vi "output check.vi"() -> ()   [LabVIEW 2012]
uses:
  <vilib>/rvi/interface/RandomDataEmulation/nirviRandomDataFPGAFIFO.vi
  <vilib>/rvi/interface/RandomDataEmulation/niFpgaRandomDataHandleErrors.vi
  <vilib>/rvi/eio/common/nirviEmuTemplateMethod_errors.vi
  <vilib>/rvi/DataTransferAndStorage/Container/XNode/niFpgaContainer.xnode
  <vilib>/rvi/interface/RandomDataEmulation/nirviRandomDataFpgaReadWriteTemplate.vi
  <vilib>/eio/EIONode/EIONode.xnode
panel:
  in  "Count(uSec)":u32
  in  "stop":bool
  out "Mod1/AI3":fxp<+/-,20,5>
  out "Mod1/AI2":fxp<+/-,20,5>
  out "Mod1/AI1":fxp<+/-,20,5>
  out "Mod1/AI0":fxp<+/-,20,5>
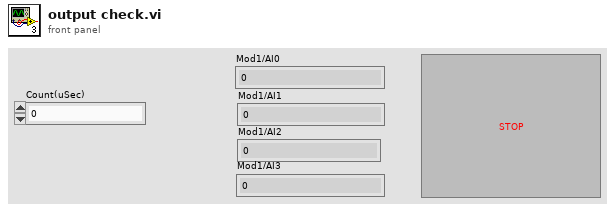
[diagram p1: front panel]
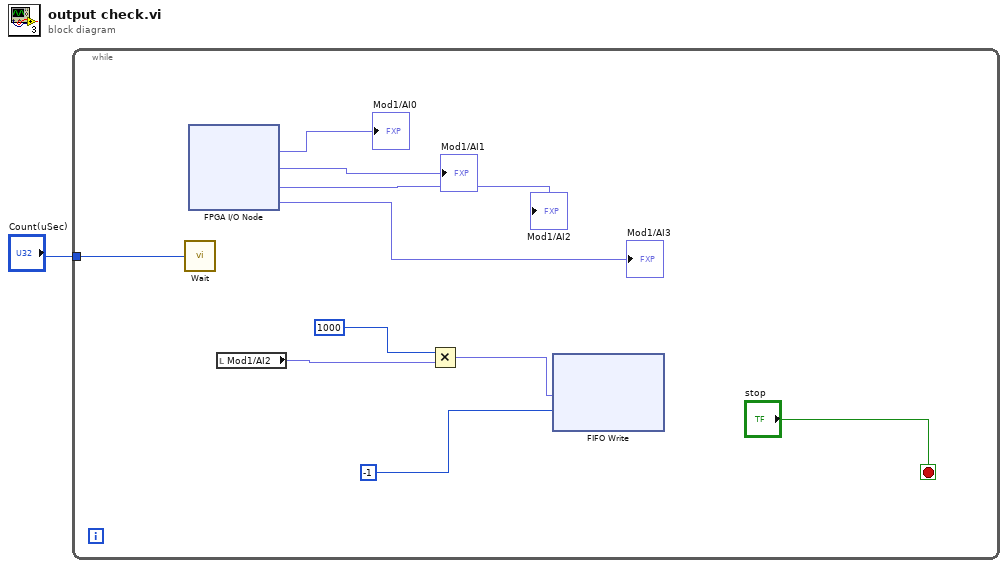
[diagram p0: block diagram]
diagram:
  n1 = while {
    tunnel: "Count(uSec)" -> [w2]
    stop <- "stop" stop-if-true
    n2 = call "Wait"("Count(uSec)"=w2) -> ()  [unwired: 1 out]
    n3 = xnode "FPGA I/O Node"() -> ("Mod1/AI0"=→"Mod1/AI0":fxp<+/-,20,5>, "Mod1/AI1"=→"Mod1/AI1":fxp<+/-,20,5>, "Mod1/AI2"=→"Mod1/AI2":fxp<+/-,20,5>, "Mod1/AI3"=→"Mod1/AI3":fxp<+/-,20,5>)  [unwired: 4 in, 4 out]
    n4 = local read "Mod1/AI2"() -> (w5:fxp<+/-,20,5>)
    n5 = Multiply(x=i64 1000, y=w5) -> (x*y=w3:fxp<+/-,64,69>)
    n6 = xnode ("FIFO Write")("Element"=w3, "Timeout"=i16 -1) -> ()  [unwired: 1 in, 2 out]
  }
